vi "2P Trigger Message Loop.vi"(8 "error in (no error)":errorcluster, 11 "Message Queues":T1) -> (0 "error out":errorcluster)   [LabVIEW 2016, in "2P Trigger.lvlib"]
doc: "The message loop subVI to handle messages pertaining to logging data."
uses:
  2P Trigger.lvlib
  support/Message Queue/All Message Queues.ctl
  support/Message Queue/Message Cluster.ctl
  2P Trigger State.ctl
  2P Trigger Config.ctl
  <vilib>/Utility/error.llb/Error Cluster From Error Code.vi
  <vilib>/ErrorRing/Error Ring.xnode
  support/Message Queue/Message Queue.lvlib
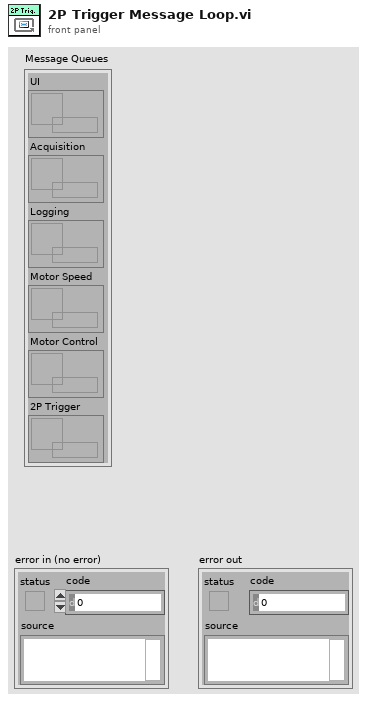
[diagram p1: front panel]
types:
  T1 = typedef "Message Queue.lvlib/All Message Queues.ctl" = cluster{"UI":refnum<queue>, "Acquisition":refnum<queue>, "Logging":refnum<queue>, "Motor Speed":refnum<queue>, "Motor Control":refnum<queue>, "2P Trigger":refnum<queue>}
  T2 = typedef "2P Trigger.lvlib/2P Trigger State.ctl" = enum16{"Idle", "Running"}
  T3 = typedef "2P Trigger.lvlib/2P Trigger Config.ctl" = cluster{"DO Line":tag}
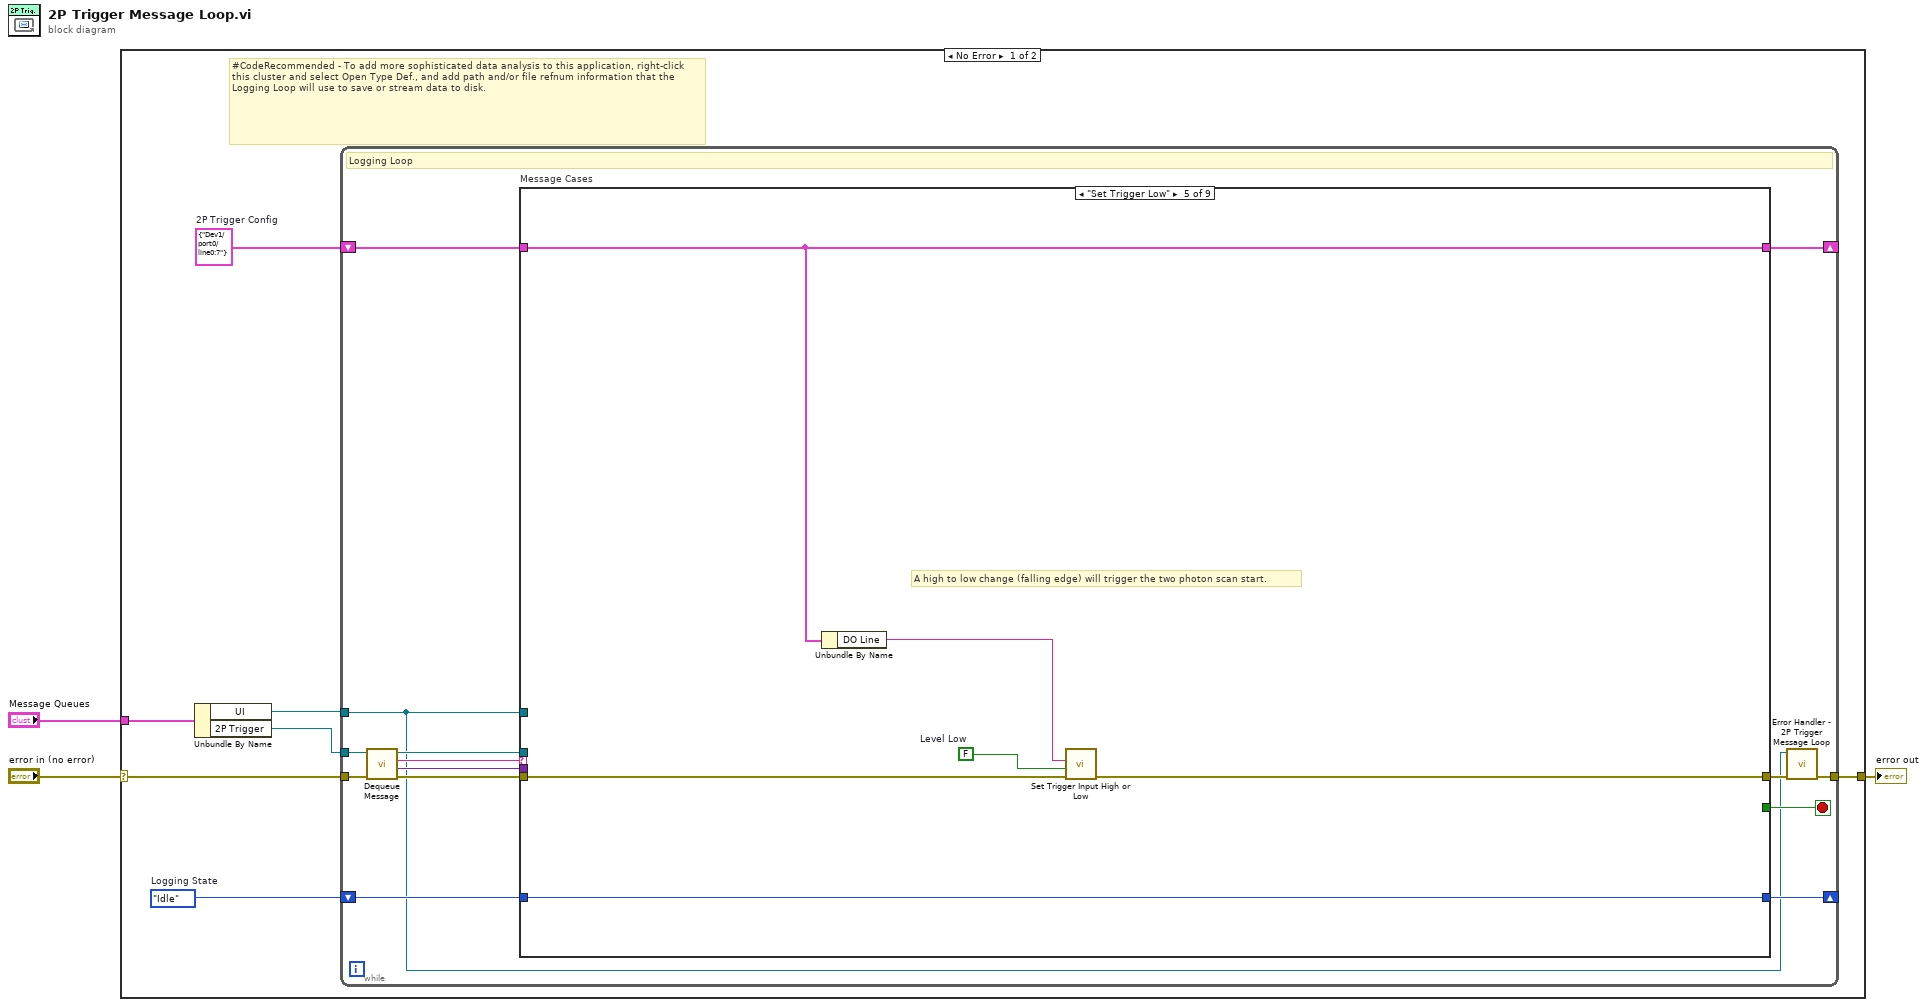
[diagram p0: block diagram]
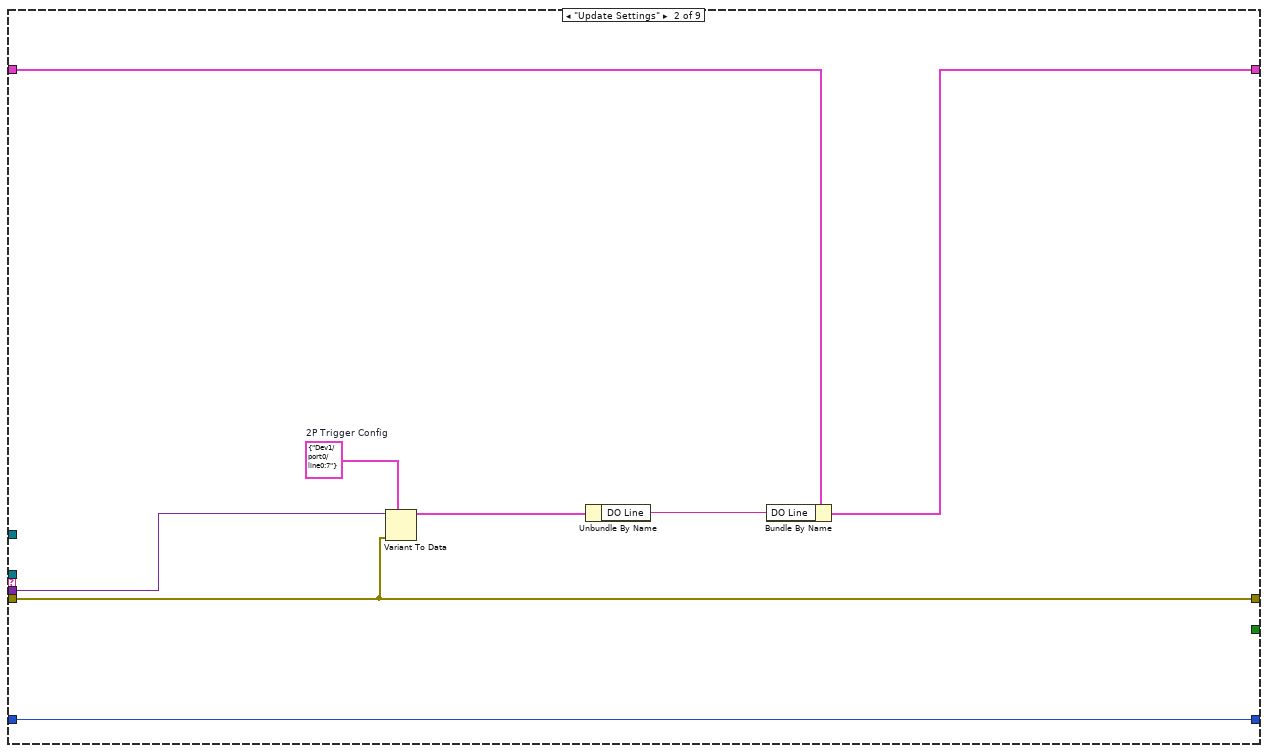
[diagram p3: hidden frame]
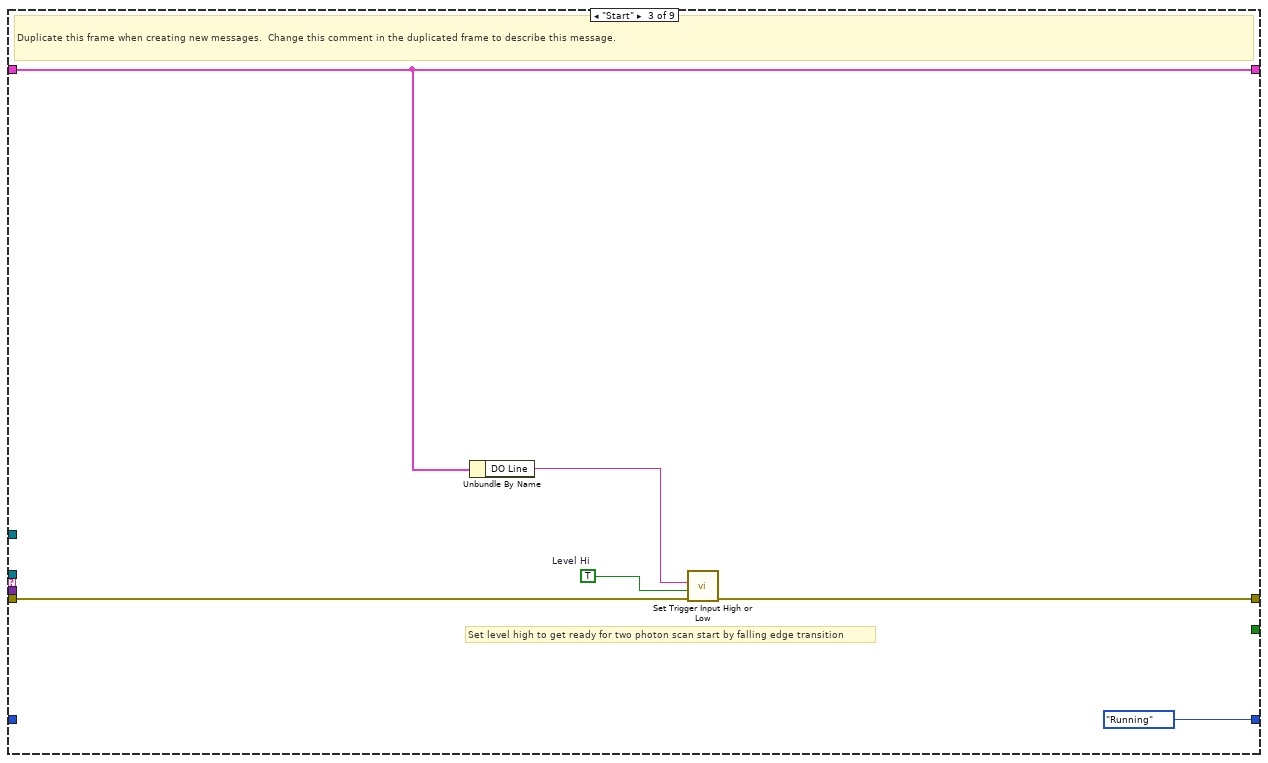
[diagram p4: hidden frame]
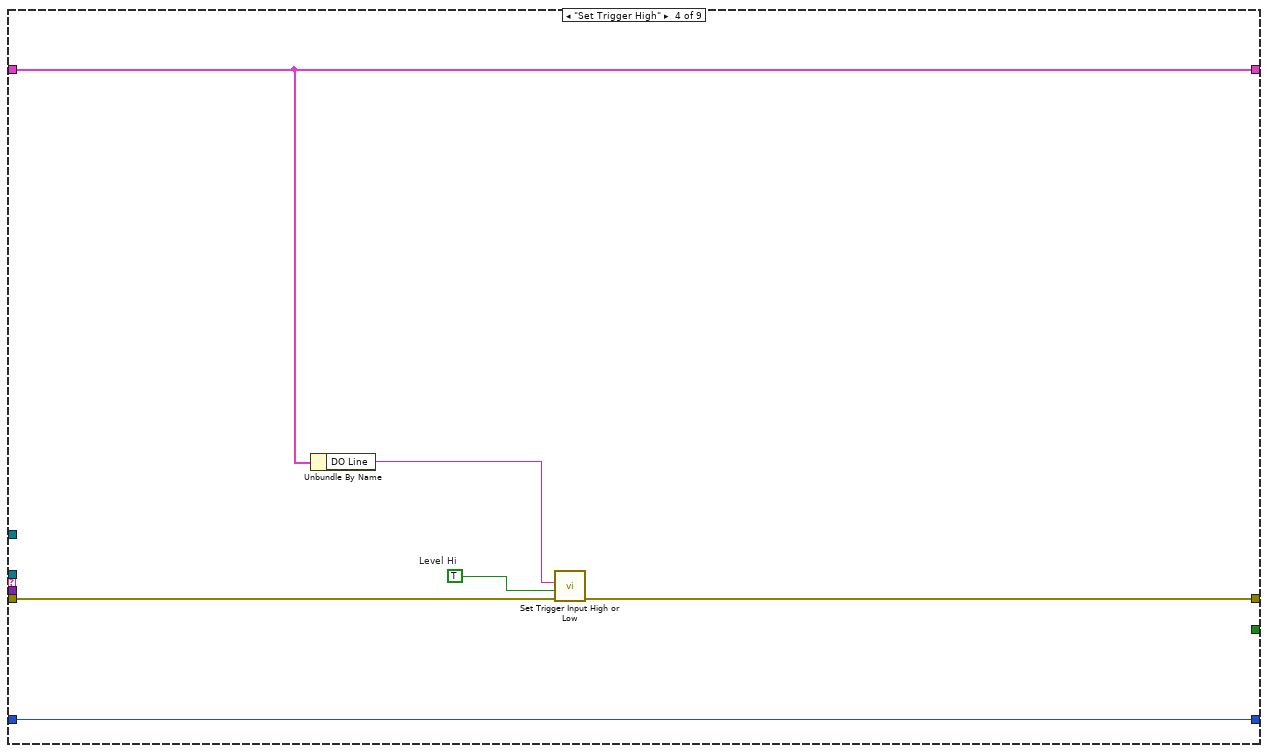
[diagram p5: hidden frame]
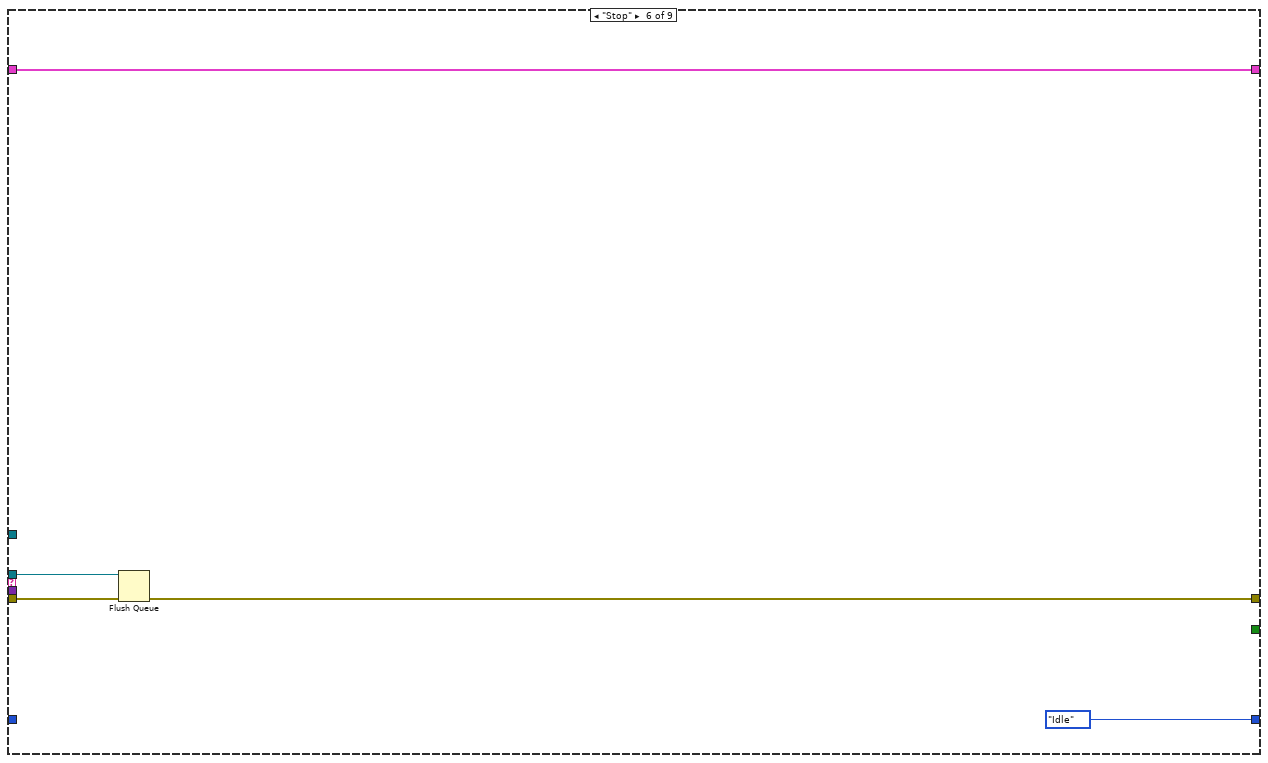
[diagram p6: hidden frame]
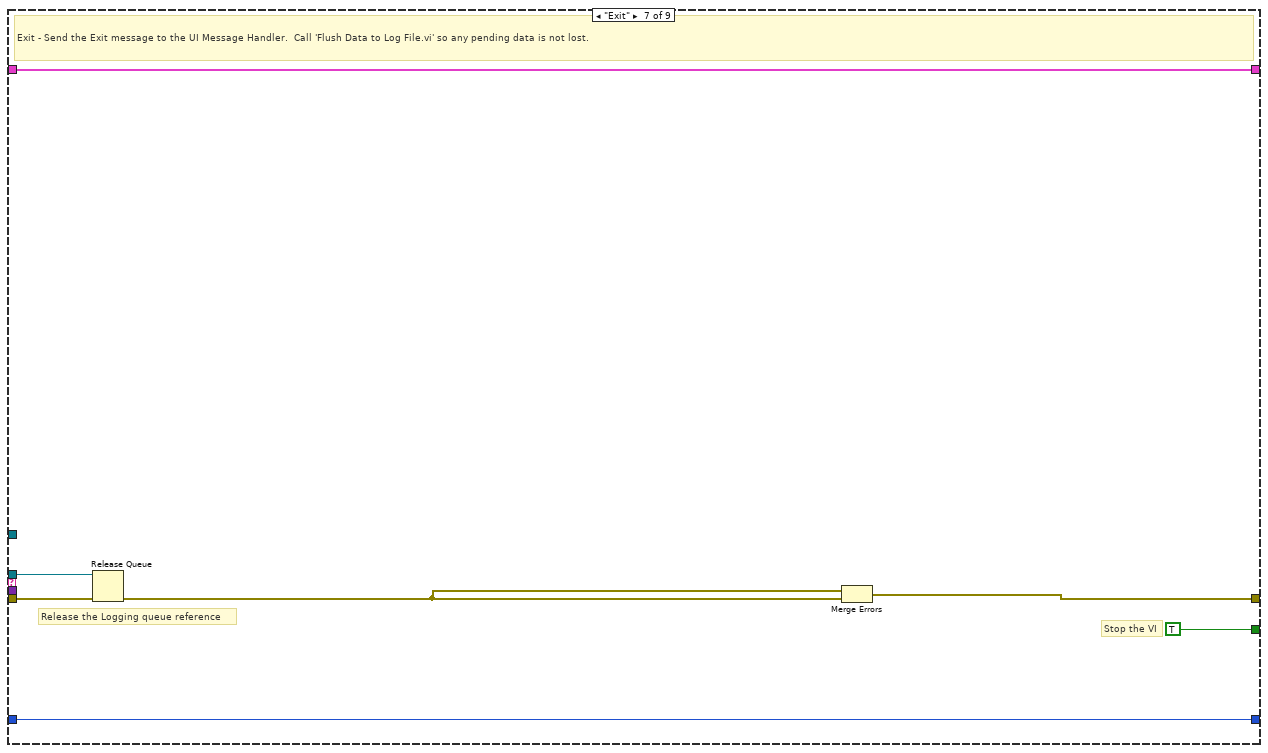
[diagram p7: hidden frame]
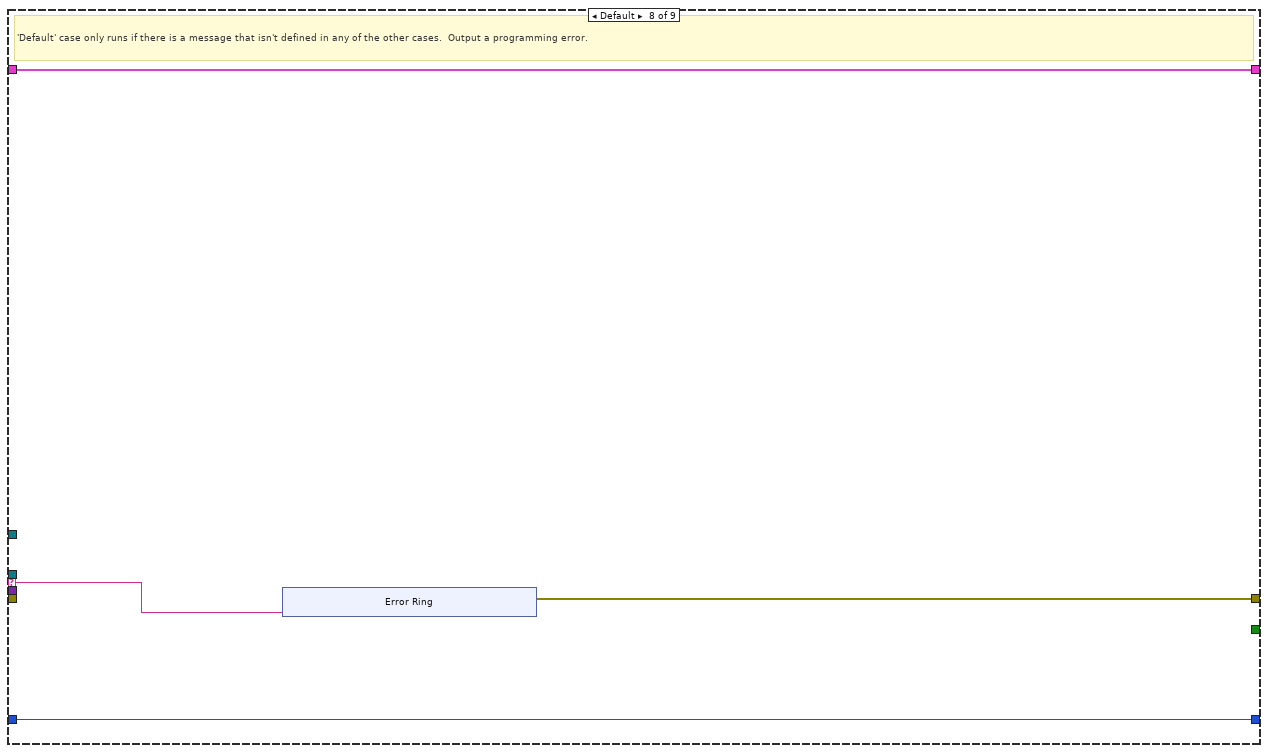
[diagram p8: hidden frame]
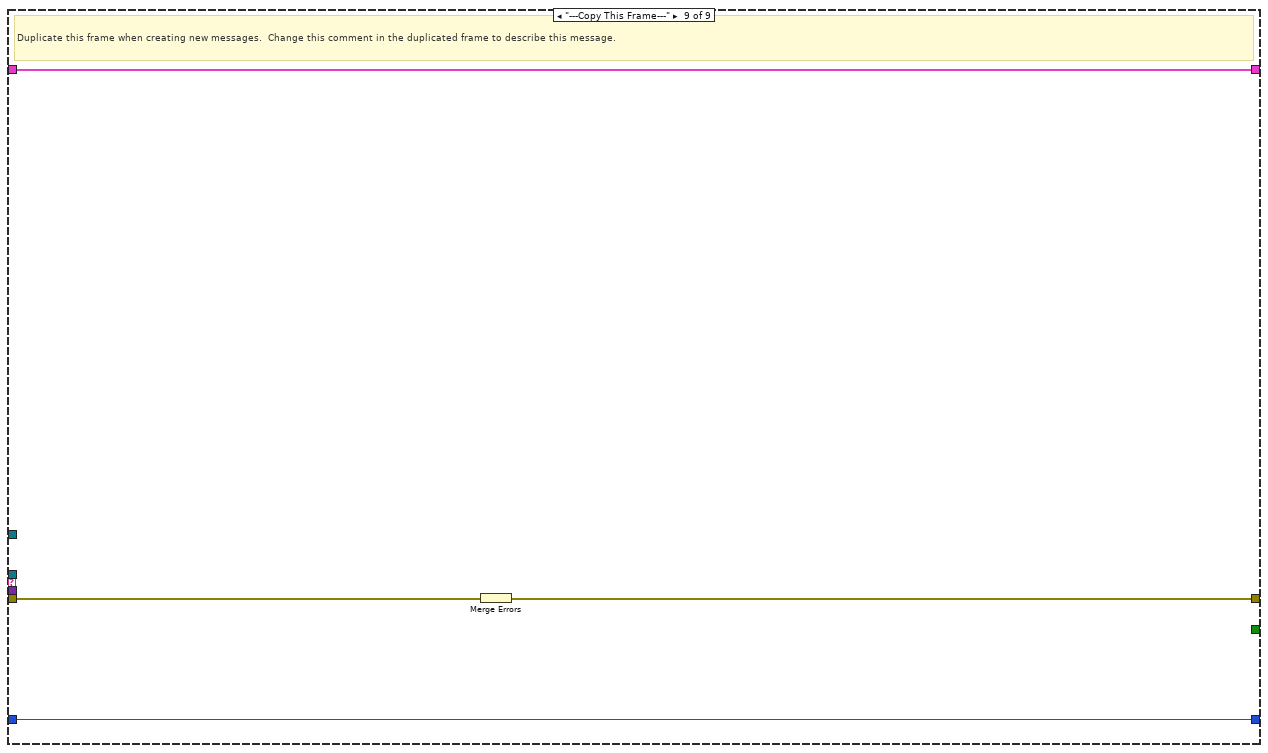
[diagram p9: hidden frame]
diagram:
  n1 = case shown="No Error" "error in (no error)" {
    selector: "error in (no error)" -> [w7 w81]
    tunnel: "Message Queues" -> [w10 _]
    tunnel: [w8 w81] -> w2
    frame No Error {
      w4 = T3 {"DO Line"="Dev1/port0/line0:7"}  # 2P Trigger Config
      w5 = 2P_Trigger_State."Idle"  # Logging State
      # "#CodeRecommended - To add more sophisticated data analysis to this application, right-click this cluster and select Open Type Def., and add path and/or file refnum information that the Logging Loop will use to save or stream data to disk."
      n2 = Unbundle By Name(w10) -> ("UI"=w6:refnum<queue>, "2P Trigger"=w9:refnum<queue>)
      n3 = while {
        tunnel: w9 -> [w16]
        shift-right: [w23] -> _
        shift-left: w4 -> [w24]
        tunnel: w6 -> [w11]
        shift-right: [w14] -> _
        shift-left: w5 -> [w15]
        tunnel: w7 -> [w21]
        tunnel: [w13] -> w8
        stop <- w22 stop-if-true
        # "Logging Loop"
        n4 = call "Dequeue Message.vi"("error in (no error)"=w21, "Message Queue"=w16) -> ("error out"=w20:errorcluster, "Message Data"=w18:variant, "Message"=w19:string, "dup Message Queue"=w17:refnum<queue>)  [unwired: 6 in]
        n5 = case "Message Cases" shown="\"Set Trigger Low\"" w19 {
          selector: w19 -> [_ _ _ _ _ _ _ w66 _]
          tunnel: w17 -> [_ _ _ _ _ w56 w62 _ _]
          tunnel: w20 -> [w26 w28 w38 w44 w50 w57 w63 _ w80]
          tunnel: [w26 w28 w37 w43 w49 w54 w64 w67 w78] -> w12
          tunnel: w24 -> [w27 w33 w40 w46 w52 w58 w60 w69 w79]
          tunnel: [w27 w32 w40 w46 w52 w58 w60 w69 w79] -> w23
          tunnel: [_ _ _ _ _ _ TRUE _ _] -> w22
          tunnel: w18 -> [_ w34 _ _ _ _ _ _ _]
          tunnel: w11 -> [_ _ _ _ _ _ _ _ _]
          tunnel: w15 -> [w25 w35 _ w47 w53 _ w61 w68 w77]
          tunnel: [w25 w35 2P_Trigger_State."Running" ("Logging State") w47 w53 2P_Trigger_State."Idle" ("Logging State") w61 w68 w77] -> w14
          frame "Initialize" {
            # "Initialize - gets called when first launched. Currently a no-op."
          }
          frame "Update Settings" {
            w30 = T3 {"DO Line"="Dev1/port0/line0:7"}  # 2P Trigger Config
            n6 = Variant To Data(error in=w28, type=w30, Variant=w34) -> (data=w31:T3)  [unwired: 1 out]
            n7 = Unbundle By Name(w31) -> ("DO Line"=w29:tag)
            n8 = Bundle By Name(cluster=w33, "DO Line"=w29) -> (w32:T3)
          }
          frame "Start" {
            w36 = TRUE  # Level Hi
            # "Set level high to get ready for two photon scan start by falling edge transition"
            # "Duplicate this frame when creating new messages.  Change this comment in the duplicated frame to describe this message."
            n9 = Unbundle By Name(w40) -> ("DO Line"=w39:tag)
            n10 = call "Set Trigger Input High or Low.vi"("error in"=w38, "Level"=w36, "Line"=w39) -> ("error out"=w37:errorcluster)  [unwired: 8 in]
          }
          frame "Set Trigger High" {
            w42 = TRUE  # Level Hi
            n11 = Unbundle By Name(w46) -> ("DO Line"=w45:tag)
            n12 = call "Set Trigger Input High or Low.vi"("error in"=w44, "Level"=w42, "Line"=w45) -> ("error out"=w43:errorcluster)  [unwired: 8 in]
          }
          frame "Set Trigger Low" {
            w48 = FALSE  # Level Low
            # "A high to low change (falling edge) will trigger the two photon scan start."
            n13 = Unbundle By Name(w52) -> ("DO Line"=w51:tag)
            n14 = call "Set Trigger Input High or Low.vi"("error in"=w50, "Level"=w48, "Line"=w51) -> ("error out"=w49:errorcluster)  [unwired: 8 in]
          }
          frame "Stop" {
            n15 = Flush Queue(queue=w56, error in (no error)=w57) -> (error out=w54:errorcluster)  [unwired: 2 out]
          }
          frame "Exit" {
            # "Release the Logging queue reference"
            # "Stop the VI"
            # "Exit - Send the Exit message to the UI Message Handler.  Call 'Flush Data to Log File.vi' so any pending data is not lost."
            n16 = Release Queue(queue=w62, error in (no error)=w63) -> (error out=w59:errorcluster)  [unwired: 1 in, 2 out]
            n17 = Merge Errors(w59, w59) -> (w64:errorcluster)
          }
          frame Default {
            # "'Default' case only runs if there is a message that isn't defined in any of the other cases.  Output a programming error."
            n18 = xnode "Error Ring"("parameter 0"=w66) -> ("error out"=w67:errorcluster)
          }
          frame "---Copy This Frame---" {
            # "Duplicate this frame when creating new messages.  Change this comment in the duplicated frame to describe this message."
            n19 = Merge Errors(w80) -> (w78:errorcluster)
          }
        }
        n20 = call "Error Handler - 2P Trigger Message Loop.vi"("error in (no error)"=w12, "Message Queue"=w11) -> ("dup error in"=w13:errorcluster)  [unwired: 8 in, 1 out]
      }
    }
    frame Error {
    }
  }
  "error out" <- w2
